vi "Make Relay JSON.vi"(9 "Force":bool, 10 "Relay prev":T1={"type"="Relay", "device"="", "name"="", "data"={"<init_fwd"=FALSE, "<init_rev"=FALSE, "<fwd"=FALSE, "<rev"=FALSE}}, 11 "Relay new":T1={"type"="Relay", "device"="", "name"="", "data"={"<init_fwd"=FALSE, "<init_rev"=FALSE, "<fwd"=FALSE, "<rev"=FALSE}}) -> (3 "delta JSON":string)   [LabVIEW 2019]
uses:
  Relay data proto.ctl
  Relay proto.ctl
panel:
  out "Complete JSON":string
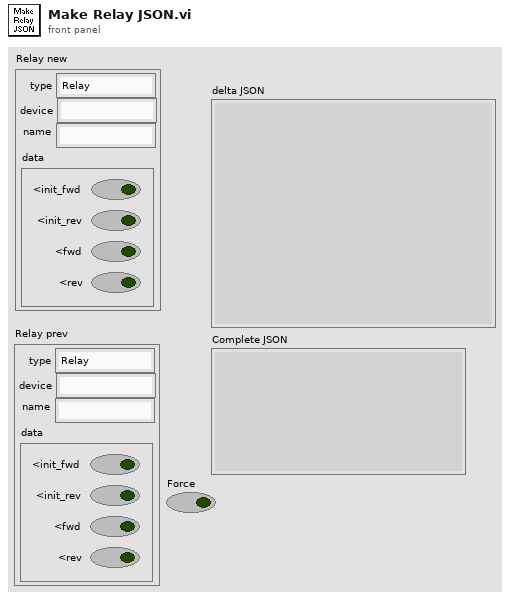
[diagram p1: front panel]
types:
  T1 = typedef "Relay proto.ctl" = cluster{"type":string, "device":string, "name":string, "data":T2}
  T2 = typedef "Relay data proto.ctl" = cluster{"<init_fwd":bool, "<init_rev":bool, "<fwd":bool, "<rev":bool}
  T3 = cluster{"type":bool, "device":bool, "name":bool, "data":T2}
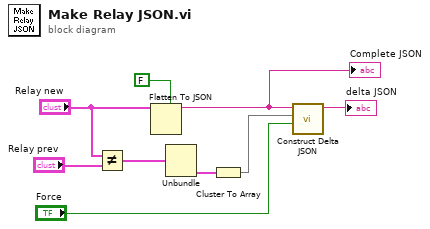
[diagram p0: block diagram]
diagram:
  n1 = Not Equal?(x="Relay new", y="Relay prev") -> (x != y?=w1:T3)
  n2 = Flatten To JSON(enable LabVIEW extensions? (T)=FALSE, anything="Relay new") -> (JSON string=w5:string)  [unwired: 1 in, 1 out]
  "Complete JSON" <- w5
  n3 = Unbundle(w1) -> ("data"=w6:T2)  [unwired: 3 out]
  n4 = Cluster To Array(cluster=w6) -> (array=w3:bool[])
  n5 = call "Construct Delta JSON.vi"("Force"="Force", "Checked Items"=w3, "JSON string"=w5) -> ("Delta JSON"=→"delta JSON":string)  [unwired: 8 in]
